vi "aaa.vi"(7 "error in":errorcluster) -> (20 "Histogram (Histogram 1)":u32[][](array[numeric]), 27 "error out":errorcluster)   [LabVIEW 2021]
panel:
  out "Image Out":T1(plugin-control)
  out "Histogram Graph":u32[][](graph)
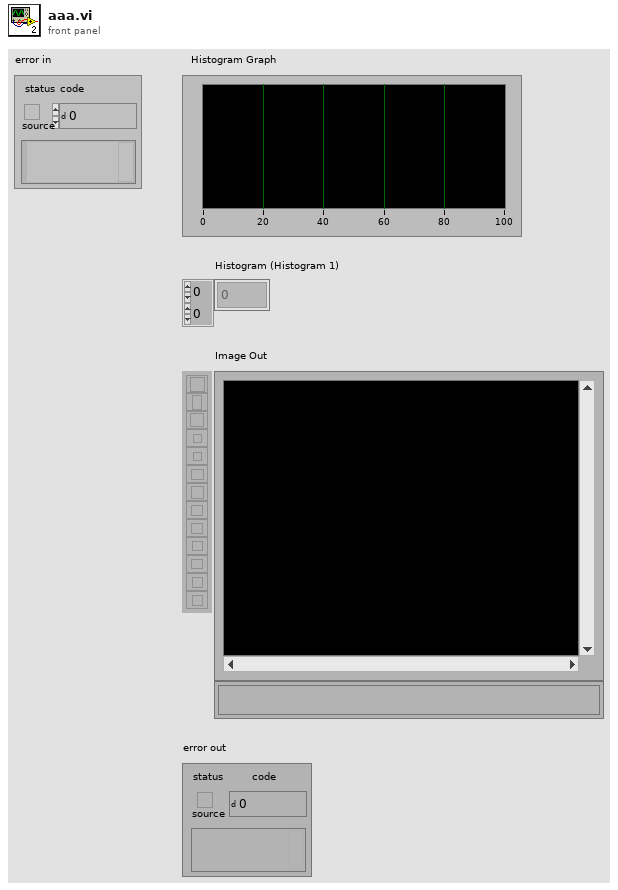
[diagram p1: front panel]
types:
  T1 = typedef "IMAQ Image.ctl" = refnum<image>
  T2 = cluster{"Global Rectangle":i32[], "Contours":cluster{"ID":enum32{"External", "Internal"}, "Type":u32, "Coordinates":i32[]}[]}
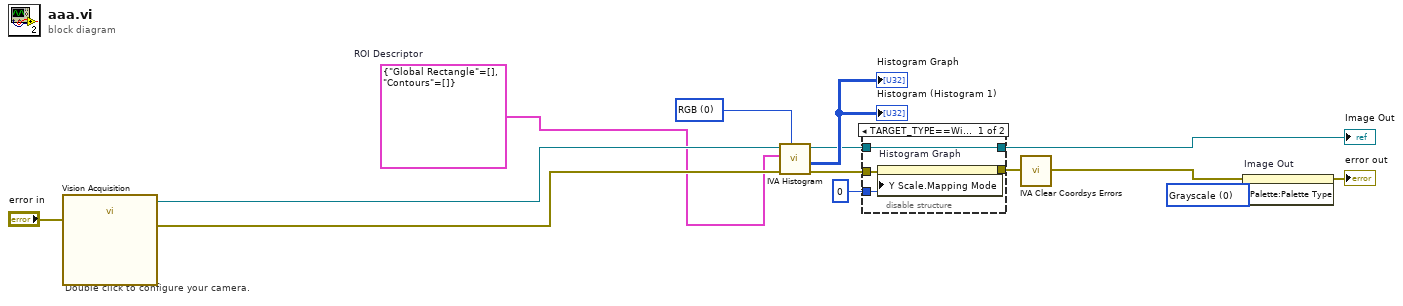
[diagram p0: block diagram]
diagram:
  w1 = u32 0 items=["Grayscale", "Binary", "Gradient", "Rainbow", "Temperature", "User Defined", "Binary 16 Bit", "Gradient 16 Bit", "Rainbow 16 Bit", "Temperature 16 Bit", "User Defined 16 Bit"] ("Palette Type")
  w10 = u16 0 items=["RGB", "HSL", "HSV", "HSI"] ("Color Mode")
  w8 = T2 {"Global Rectangle"=[], "Contours"=[]}  # ROI Descriptor
  # "Double click to configure your camera."
  n1 = call "Vision Acquisition"("error in"="error in") -> ("Image Out"=w12:T1, "error out"=w13:errorcluster)  [unwired: 25 in]
  n2 = call <vilib>:"IVA Histogram.vi"("Color Mode"=w10, "error in (no error)"=w13, "ROI Descriptor"=w8, "Image In"=w12) -> ("error out"=w11:errorcluster, "Histograms"=→"Histogram Graph" →"Histogram (Histogram 1)":u32[][], "Image Out"=w7:T1)  [unwired: 5 out]
  n3 = disable-structure "조건적 비활성화 구조" shown="TARGET_TYPE==Windows" {
    disable-tunnel: w11 -> [w18 w19]
    disable-tunnel: [w17 w19] -> w5
    disable-tunnel: w7 -> [w16 w20]
    disable-tunnel: [w16 w20] -> w2
    disable-tunnel: u8 0 ("Y Scale.Mapping Mode") -> [w15 _]
    frame condition #0 (active) {
      n4 = property on="Histogram Graph" class="WFGraph (엄격한)"(error in=w18, "Y Scale.Mapping Mode"=w15) -> (error out=w17:errorcluster)  [unwired: 1 in, 1 out]
    }
    frame condition #1 {
    }
  }
  "Image Out" <- w2
  n5 = call <vilib>:"IVA Clear Coordsys Errors.vi"("error in (no error)"=w5) -> ("error out"=w4:errorcluster)  [unwired: 10 in]
  n6 = property on="Image Out" class="ImageControl"(error in=w4, "Palette:Palette Type"=w1) -> (error out=→"error out":errorcluster)  [unwired: 1 in, 1 out]
